vi "Create_RFID_Baseband small_CW.vi"(5 "Parameters Symbols":T1={"Tari"=8e-06, "PW"=0.5, "factor for \"1\" symbol"=0.5, "RTcal"=2.5, "TRcal"=3.0, "Delimiter"=1.25e-05} {"TRcal" min=1.1 max=3.0 step=0.1; "RTcal" min=2.5 max=3.0 step=0.1; "factor for \"1\" symbol" min=0.5 max=1.0 step=0.1; "PW" min=0.265 max=0.525 step=0.001; "Tari" format="%#_3p"}, 9 "Symbol Rate [Hz]":dbl, 11 "error in":errorcluster) -> (6 "complex waveform":cluster{"t0":dbl, "dt":dbl, "Y":cdb[]}, 15 "error out":errorcluster)   [LabVIEW 2015]
uses:
  <vilib>/addons/Modulation/Analog/support/mod_Set Error Source.vi
  <vilib>/addons/Modulation/Digital/General/MT Generate ASK system parameters (M).vi
  <vilib>/addons/Modulation/Digital/Support/Common/Validators/mod_Generate Filter Coefficients Validate.vi
  <vilib>/addons/Modulation/Digital/General/subVIs/mod_Generate Filter Coefficients.vi
  <vilib>/addons/Modulation/niDMT.lvlib
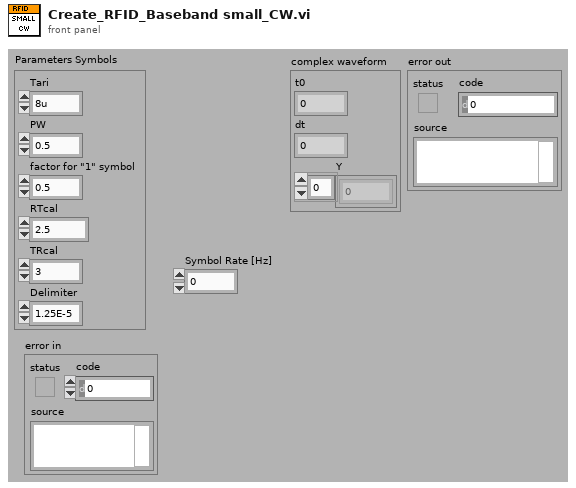
[diagram p1: front panel]
types:
  T1 = cluster{"Tari":dbl, "PW":dbl, "factor for \"1\" symbol":dbl, "RTcal":dbl, "TRcal":dbl, "Delimiter":dbl}
  T2 = enum16{"none", "Raised Cosine", "Root Raised Cos", "Gaussian"}
  T3 = cluster{"samples per symbol (16)":i32, "symbol map":cdb[]}
  T4 = typedef "niAMT.lvlib/Complex Data Waveform.ctl" = cluster{"t0":dbl, "dt":dbl, "Y":cdb[]}
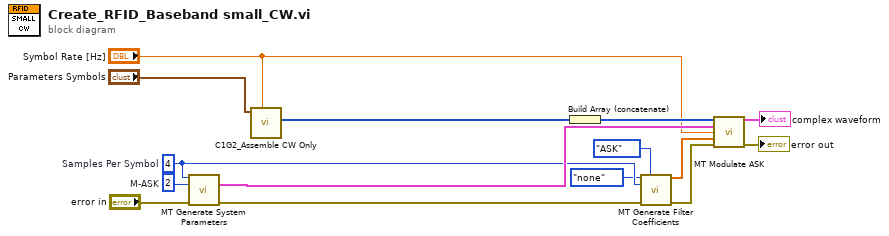
[diagram p0: block diagram]
diagram:
  w10 = 2  # M-ASK
  w6 = 4  # Samples Per Symbol
  n1 = call-poly <vilib>:"MT Generate System Parameters.vi"("samples per symbol (16)"=w6, "M-ASK (2)"=w10, "error in (no error)"="error in") -> ("ASK system parameters"=w11:T3, "error out"=w8:errorcluster)  [unwired: 10 in, 1 out]
  n2 = call "C1G2_Assemble CW Only.vi"("Symbol Rate"="Symbol Rate [Hz]", "Parameters Symbols"="Parameters Symbols") -> ("Signal out"=w3:u8[])  [unwired: 9 in]
  n3 = Build Array (concatenate)(w3) -> (w4:u8[])
  n4 = call <vilib>:"MT Generate Filter Coefficients.vi"("pulse shaping filter (none)"=T2."none", "modulation type"=enum16{"FSK", "PSK", "QAM", "MSK", "PAM", "ASK"}."ASK", "pulse shaping samples per symbol (16)"=w6, "error in (no error)"=w8) -> ("pulse shaping filter coefficients"=w12:dbl[], "error out"=w7:errorcluster)  [unwired: 9 in, 1 out]
  n5 = call <vilib>:"MT Modulate ASK.vi"("input bit stream"=w4, "ASK system parameters"=w11, "symbol rate (Hz)"="Symbol Rate [Hz]", "pulse shaping filter coefficients"=w12, "error in (no error)"=w7) -> ("output complex waveform"=→"complex waveform":T4, "error out"=→"error out":errorcluster)  [unwired: 8 in, 1 out]
